vi "SoftFrontPanel.vi"(8 "error in":errorcluster, 11 "PS Instrument":refnum<class "Power Supply Instrument.lvclass">) -> (0 "error out":errorcluster, 3 "PS Instrument out":refnum<class "Power Supply Instrument.lvclass">)   [LabVIEW 2025, in "Power Supply.lvlib" / "Power Supply Instrument.lvclass"]
doc: "Copyright 2017 National Instruments Corporation\n\nLicensed under the Apache License, Version 2.0 (the \"License\"); you may not use this file except in compliance with the License. You may obtain a copy of the License at http://www.apache.org/licenses/LICENSE-2.0\nUnless required by applicable law or agreed to in writing, software distributed under the License is distributed on an \"AS IS\" BASIS, WITHOUT WARRANTIES OR CONDITIONS OF ANY KIND, either express or implied. See the License for the specific language governing permissions and limitations under the License."
uses:
  Power Supply Instrument.lvclass
  Power Supply Instrument.lvclass/Power Supply Instrument.ctl
  Users/Public/Documents/Sandia National Labs/TSS Plugin/Abstract Engine.lvlibp/Instrument configuration/Instrument configuration.lvclass
panel:
  in  "output":bool
  in  "ChannelBTN":enum32{"Ch0", "Ch1", "Ch2", "Ch3"}(radio)
  out "SFP":T1={"Chname"="Ch0", "Voltage"=0.0, "Current"=0.0} {"Voltage" format="%#_6f"; "Current" format="%#_6f"}
  out "Instrument":string caption="Instrument ::"
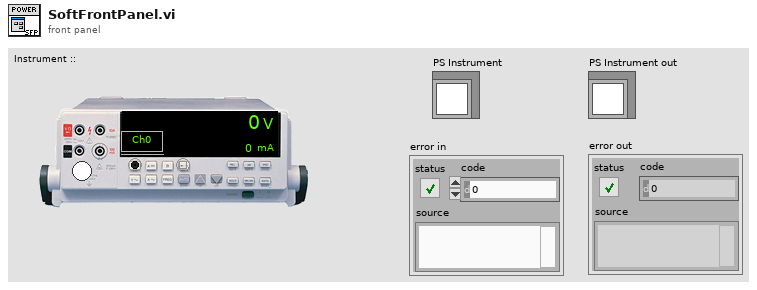
[diagram p1: front panel]
types:
  T1 = cluster{"Chname":string, "Voltage":dbl, "Current":dbl}
  T2 = enum32{"Invalid", "Default", "Floating", "Floating/Auto-Hide", "Modal"}
  T3 = typedef "Abstract Engine.lvlibp/Instrument configuration.lvclass/Default Instrument.ctl" = cluster{"Type":string, "Address":string, "SW Alias":string, "Description":string, "Enabled":bool}
  T4 = cluster{"Channel":string, "Voltage":dbl, "Current":dbl}
  T5 = typedef "Abstract Engine.lvlibp/Abstract Instrument.lvclass/Channel.ctl" = cluster{"Alias":string, "DataType":enum16{"Anaolg Input", "Waveform"}, "Unit":enum16{"---", "V", "A", "Ohm", "Hz", "uF", "degC", "deg"}, "Upper limit":dbl, "Lower limit":dbl, "Measurement":variant}
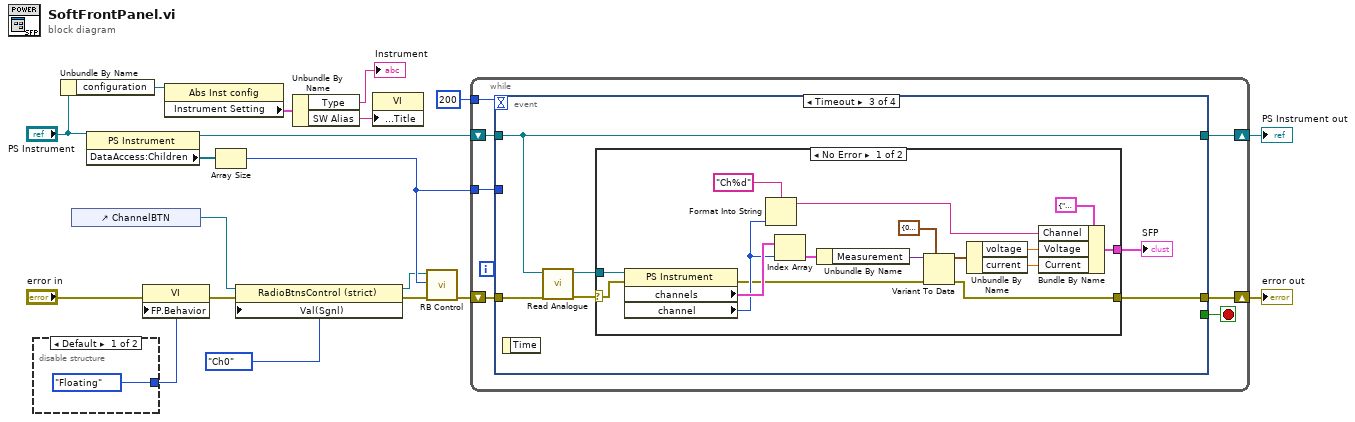
[diagram p0: block diagram]
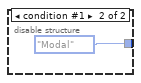
[diagram p2: hidden frame]
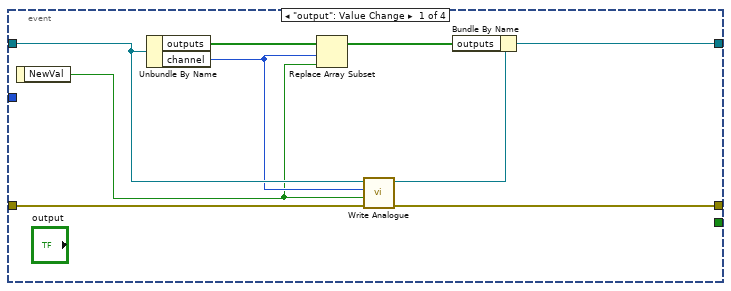
[diagram p3: hidden frame]
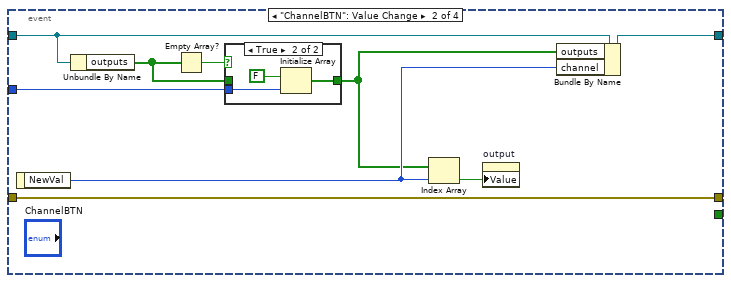
[diagram p4: hidden frame]
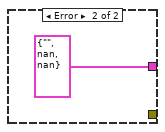
[diagram p6: hidden frame]
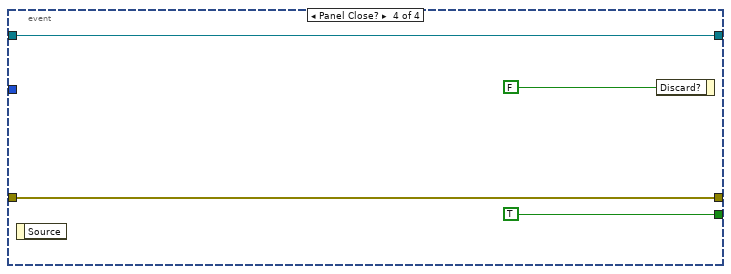
[diagram p7: hidden frame]
diagram:
  n1 = disable-structure shown="Default" {
    disable-tunnel: [T2."Floating" ("Front Panel Window:Behavior") T2."Modal" ("Front Panel Window:Behavior")] -> w15
    frame condition #0 (active) {
    }
    frame condition #1 {
    }
  }
  n2 = Unbundle By Name("PS Instrument") -> ("configuration"=w19:refnum<class "Instrument configuration.lvclass">)
  n3 = control-ref of="ChannelBTN"() -> (w3:refnum<vi>)
  n4 = property class="PS Instrument"(reference="PS Instrument") -> (reference out=w6:refnum<class "Power Supply Instrument.lvclass">, "DataAccess:Children"=w7:refnum<data-value>[])  [unwired: 1 in, 1 out]
  n5 = property class="VI"(error in="error in", "FP.Behavior"=w15) -> (error out=w8:errorcluster)  [unwired: 1 in, 1 out]
  n6 = property class="Abs Inst config"(reference=w19) -> ("Instrument Setting"=w18:T3)  [unwired: 1 in, 2 out]
  n7 = Array Size(array=w7) -> (size(s)=w5:i32)
  n8 = property class="RadioBtnsControl (strict)"(reference=w3, error in=w8, "Val(Sgnl)"=enum32{"Ch0", "Ch1", "Ch2", "Ch3"}."Ch0" ("Value (Signaling)")) -> (reference out=w2:refnum<vi>, error out=w4:errorcluster)
  n9 = Unbundle By Name(w18) -> ("Type"=→"Instrument":string, "SW Alias"=w17:string)
  n10 = property class="VI"("Front Panel.Title"=w17) -> ()  [unwired: 2 in, 2 out]
  n11 = call "RB Control.vi"("error in"=w4, "Channels"=w5, "Radio Ref"=w2) -> ("error out"=w14:errorcluster)  [unwired: 8 in]
  n12 = while {
    shift-right: [w26] -> w13
    shift-left: w14 -> [w27]
    shift-right: [w24] -> w12
    shift-left: w6 -> [w25]
    tunnel: 200 -> [w23]
    tunnel: w5 -> [w22]
    stop <- w28 stop-if-true
    n13 = event shown="[2] Timeout" {
      selector: _ -> [_ _ _ _]
      dyn-events: _ -> [_ _ _ _]
      timeout: w23 -> [_ _ _ _]
      tunnel: [_ _ _ TRUE] -> w28
      tunnel: [w37 w44 w55 w75] -> w26
      tunnel: w27 -> [w36 w44 w52 w75]
      tunnel: w25 -> [w34 w46 w54 w74]
      tunnel: [w33 w45 w54 w74] -> w24
      tunnel: w22 -> [_ w39 _ _]
      event "output": Value Change {
        n14 = event-data() -> ("NewVal"=w29:bool)  [unwired: 1 in]
        n15 = Unbundle By Name(w34) -> ("outputs"=w32:bool[], "channel"=w30:enum32{"Ch0", "Ch1", "Ch2", "Ch3"})
        n16 = Replace Array Subset(array=w32, new element=w29, index=w30) -> (w31:bool[])
        n17 = call-dynamic "Write Analogue.vi"("error in (no error)"=w36, "output"=w29, "Channel index"=w30, "PS Instrument"=w34) -> ("error out"=w37:errorcluster, "PS Instrument out"=w35:refnum<class "Power Supply Instrument.lvclass">)  [unwired: 5 in, 1 out]
        n18 = Bundle By Name(cluster=w35, "outputs"=w31) -> (w33:refnum<class "Power Supply Instrument.lvclass">)
      }
      event "ChannelBTN": Value Change {
        n19 = event-data() -> ("NewVal"=w42:enum32{"Ch0", "Ch1", "Ch2", "Ch3"})  [unwired: 1 in]
        n20 = Unbundle By Name(w46) -> ("outputs"=w40:bool[])
        n21 = Empty Array?(array=w40) -> (empty?=w41:bool)
        n22 = case shown="True" w41 {
          tunnel: w40 -> [w47 _]
          tunnel: w39 -> [_ w49]
          tunnel: [w47 w48] -> w38
          frame False {
          }
          frame True {
            n23 = Initialize Array(FALSE, w49) -> (w48:bool[])
          }
        }
        n24 = Index Array(array=w38, index=w42) -> (element=w43:bool)
        n25 = property on="output" class="Bool (strict)"("Value"=w43) -> ()  [unwired: 2 in, 2 out]
        n26 = Bundle By Name(cluster=w46, "outputs"=w38, "channel"=w42) -> (w45:refnum<class "Power Supply Instrument.lvclass">)
      }
      event Timeout {
        n27 = event-data() -> ()  [unwired: 1 in, 1 out]
        n28 = call-dynamic "Read Analogue.vi"("error in (no error)"=w52, "PS Instrument"=w54) -> ("error out"=w51:errorcluster, "PS Instrument out"=w53:refnum<class "Power Supply Instrument.lvclass">)  [unwired: 7 in, 1 out]
        n29 = case shown="No Error" w51 {
          selector: w51 -> [w57 _]
          tunnel: [w71 T4 {"Channel"="", "Voltage"=nan, "Current"=nan} ("DataSet")] -> w56
          tunnel: [w59 _] -> w55
          tunnel: w53 -> [w58 _]
          frame No Error {
            n30 = property class="PS Instrument"(reference=w58, error in=w57) -> (error out=w60:errorcluster, "channels"=w66:T5[], "channel"=w61:enum32{"Ch0", "Ch1", "Ch2", "Ch3"})  [unwired: 1 out]
            n31 = Format Into String(format string="Ch%d", w61) -> (resulting string=w62:string)  [unwired: 2 in, 1 out]
            n32 = Index Array(array=w66, index=w61) -> (element=w68:T5)
            n33 = Unbundle By Name(w68) -> ("Measurement"=w65:variant)
            n34 = Variant To Data(error in=w60, type=cluster{"voltage":dbl, "current":dbl} {"voltage"=0.0, "current"=0.0} ("output cluster"), Variant=w65) -> (data=w63:cluster{"voltage":dbl, "current":dbl}, error out=w59:errorcluster)
            n35 = Unbundle By Name(w63) -> ("voltage"=w70:dbl, "current"=w69:dbl)
            n36 = Bundle By Name(cluster=T4 {"Channel"="", "Voltage"=0.0, "Current"=0.0} ("DataSet"), "Channel"=w62, "Voltage"=w70, "Current"=w69) -> (w71:T4)
          }
          frame Error {
          }
        }
        "SFP" <- w56
      }
      event Panel Close? {
        n37 = event-data() -> ()  [unwired: 1 in, 1 out]
        n38 = event-data("Discard?"=FALSE) -> ()  [unwired: 1 in, 1 out]
      }
    }
  }
  "error out" <- w13
  "PS Instrument out" <- w12
